vi "Get X Y Ratios.vi"(11 "Facing":dbl) -> (2 "Y Ratio":dbl, 3 "X Ratio":dbl)   [LabVIEW 2015]
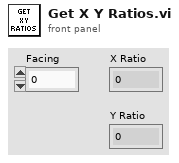
[diagram p1: front panel]
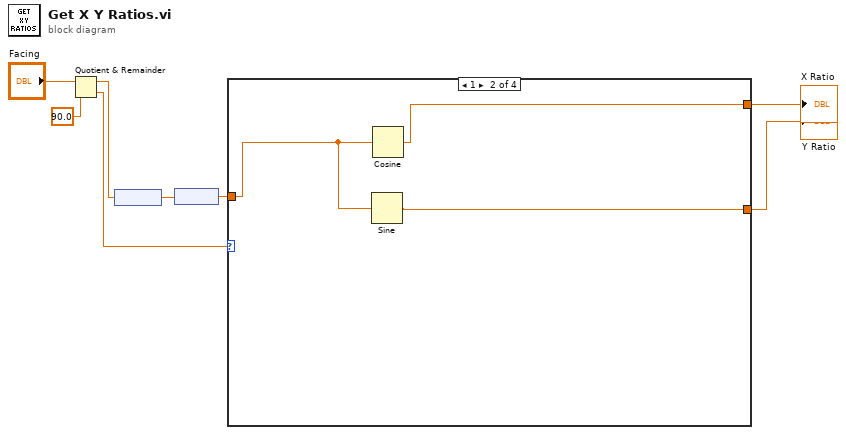
[diagram p0: block diagram]
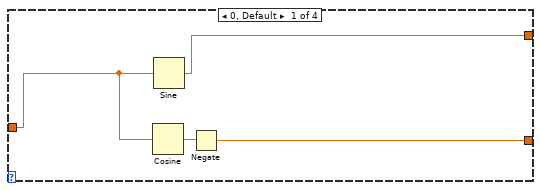
[diagram p2: hidden frame]
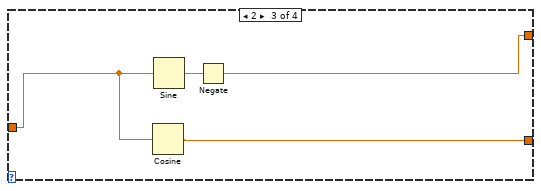
[diagram p3: hidden frame]
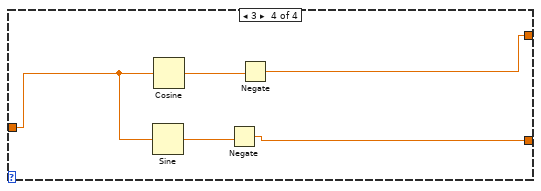
[diagram p4: hidden frame]
diagram:
  n1 = Quotient & Remainder(x="Facing", y=90.0) -> (x-y*floor(x/y)=w5:dbl, floor(x/y)=w3:dbl)
  n2 = node(w5) -> (w4:dbl[unit])
  n3 = node(w4) -> (w6:dbl)
  n4 = case shown="1" w3 {
    tunnel: w6 -> [w12 w15 w19 w24]
    tunnel: [w10 w13 w18 w22] -> w7
    tunnel: [w9 w14 w16 w20] -> w8
    frame 0, Default {
      n5 = Cosine(x=w12) -> (cos(x)=w11:dbl)
      n6 = Sine(x=w12) -> (sin(x)=w9:dbl)
      n7 = Negate(x=w11) -> (-x=w10:dbl)
    }
    frame 1 {
      n8 = Sine(x=w15) -> (sin(x)=w13:dbl)
      n9 = Cosine(x=w15) -> (cos(x)=w14:dbl)
    }
    frame 2 {
      n10 = Cosine(x=w19) -> (cos(x)=w18:dbl)
      n11 = Sine(x=w19) -> (sin(x)=w17:dbl)
      n12 = Negate(x=w17) -> (-x=w16:dbl)
    }
    frame 3 {
      n13 = Sine(x=w24) -> (sin(x)=w23:dbl)
      n14 = Cosine(x=w24) -> (cos(x)=w21:dbl)
      n15 = Negate(x=w23) -> (-x=w22:dbl)
      n16 = Negate(x=w21) -> (-x=w20:dbl)
    }
  }
  "X Ratio" <- w8
  "Y Ratio" <- w7
